vi "Read DUMMY.vi"(8 "error in (no error)":errorcluster, 11 "Instance Handle":T1) -> (0 "error out":errorcluster, 2 "DUMMY":bool, 3 "Session Handle Out":T1)   [LabVIEW 2011, in "Singleton.lvclass"]
uses:
  Singleton.lvclass
  Typedefs/Instance handle.ctl
  Singleton.lvclass/Singleton.ctl
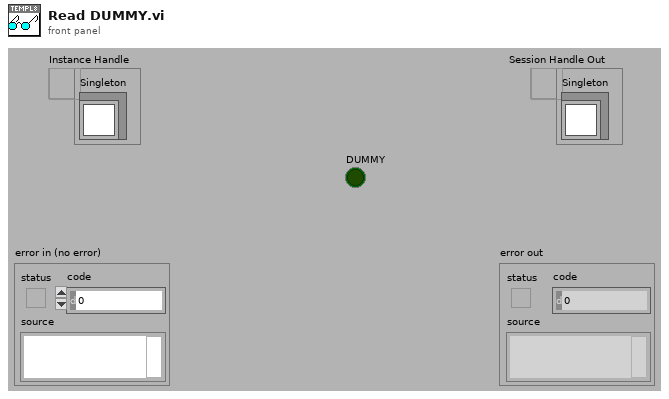
[diagram p1: front panel]
types:
  T1 = typedef "Singleton.lvclass/Instance handle.ctl" = refnum<data-value>
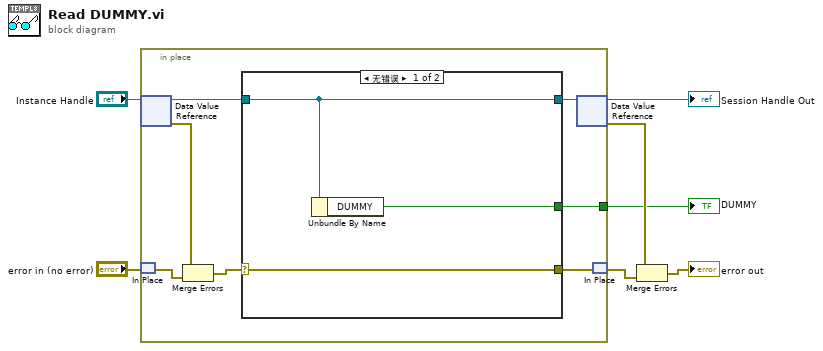
[diagram p0: block diagram]
diagram:
  n1 = in-place {
    in-place-border: [w8] -> w1
    n2 = in-place-dvr #1("Instance Handle") -> (w10:refnum<class "Singleton.lvclass">, w11:errorcluster)
    n3 = in-place-match #2("error in (no error)") -> (w12:errorcluster)
    n4 = Merge Errors(w11, w12) -> (w14:errorcluster)
    n5 = case shown="无错误" w14 {
      selector: w14 -> [w17 w18]
      tunnel: [w17 w18] -> w13
      tunnel: w10 -> [w16 w19]
      tunnel: [w16 w19] -> w9
      tunnel: [w15 _] -> w8
      frame No Error {
        n6 = Unbundle By Name(w16) -> ("DUMMY"=w15:bool)
      }
      frame Error {
      }
    }
    n7 = in-place-dvr #1(w9) -> (→"Session Handle Out":T1, w3:errorcluster)
    n8 = in-place-match #2(w13) -> (w2:errorcluster)
  }
  "DUMMY" <- w1
  n9 = Merge Errors(w3, w2) -> (→"error out":errorcluster)
